vi "Setup SMU_PD and Measure Capacitance Only - Copy.vi"(0 "Semiconductor Module Context":T2, 1 "SMU_PD_Pin":string[](array[string])=["VDD"], 2 "Measurement Id":string="CMax", 3 "PD_v":dbl=41.0 format="%#_13g", 5 "error in (no error)":errorcluster, 6 "VNAs Measurement Parameters":T1) -> (14 "Semiconductor Module Context Out":T2, 19 "error out":errorcluster)   [LabVIEW 2013]
uses:
  <vilib>/NI_TestStand_SemiconductorModule/NI_TestStand_Semiconductor_Module.lvlibp/PinMap/General/SemiconductorModuleContext.ctl
  VNA/VNAs Measurement Parameters.ctl
  <vilib>/NI_TestStand_SemiconductorModule/NI_TestStand_Semiconductor_Module.lvlibp
panel:
  in  "SMU_PD_PU_v":dbl=1.8 caption="voltage level" format="%_6p"
  in  "SMU_PD_PU_Pin":string[](array[string])=["VDD"]
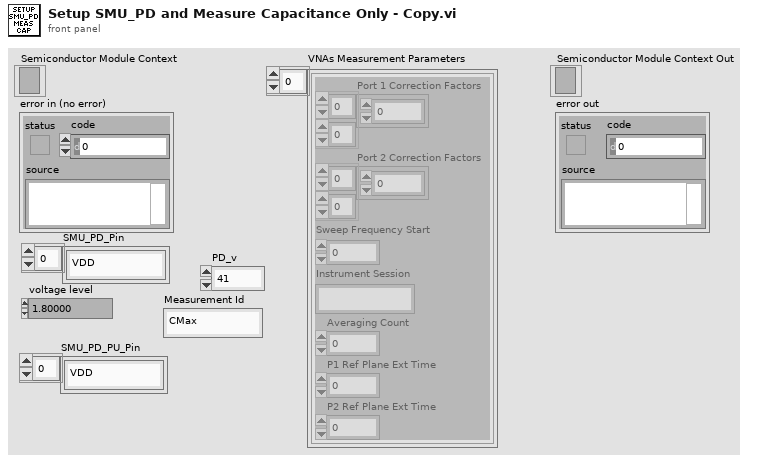
[diagram p1: front panel]
types:
  T1 = typedef "VNAs Measurement Parameters.ctl" = cluster{"Port 1 Correction Factors":cdb[][], "Port 2 Correction Factors":cdb[][], "Sweep Frequency Start":dbl, "Instrument Session":string, "Averaging Count":i32, "P1 Ref Plane Ext Time":dbl, "P2 Ref Plane Ext Time":dbl}[]
  T2 = typedef "NI_TestStand_Semiconductor_Module.lvlibp/SemiconductorModuleContext.ctl" = refnum<k7>
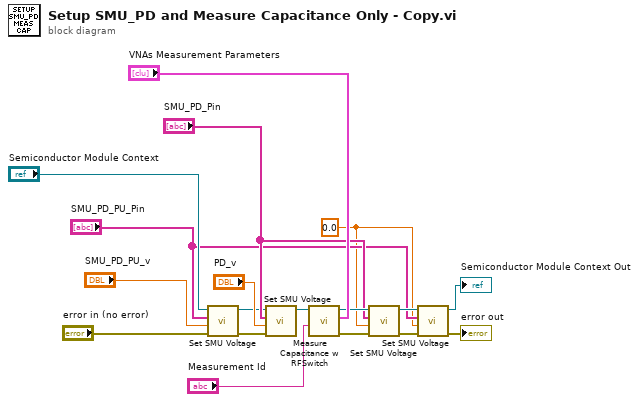
[diagram p0: block diagram]
diagram:
  w1 = 0.0 ("VDD voltage level")
  n1 = call "Set SMU Voltage.vi"("error in (no error)"="error in (no error)", "VDD voltage level"="SMU_PD_PU_v", "Pins"="SMU_PD_PU_Pin", "Semiconductor Module Context"="Semiconductor Module Context") -> ("error out"=w10:errorcluster, "Semiconductor Module Context Out"=w6:T2)  [unwired: 5 in, 1 out]
  n2 = call "Set SMU Voltage.vi"("error in (no error)"=w10, "VDD voltage level"="PD_v", "Pins"="SMU_PD_Pin", "Semiconductor Module Context"=w6) -> ("Semiconductor Module Context Out"=w12:T2)  [unwired: 5 in, 2 out]
  n3 = call "Measure Capacitance w RFSwitch.vi"("VNAs Measurement Parameters"="VNAs Measurement Parameters", "Measurement Id"="Measurement Id", "Semiconductor Module Context"=w12) -> ("error out"=w13:errorcluster, "Semiconductor Module Context Out"=w15:T2)  [unwired: 6 in, 1 out]
  n4 = call "Set SMU Voltage.vi"("error in (no error)"=w13, "VDD voltage level"=w1, "Pins"="SMU_PD_Pin", "Semiconductor Module Context"=w15) -> ("error out"=w9:errorcluster, "Semiconductor Module Context Out"=w5:T2)  [unwired: 5 in, 1 out]
  n5 = call "Set SMU Voltage.vi"("error in (no error)"=w9, "VDD voltage level"=w1, "Pins"="SMU_PD_PU_Pin", "Semiconductor Module Context"=w5) -> ("error out"=→"error out":errorcluster, "Semiconductor Module Context Out"=→"Semiconductor Module Context Out":T2)  [unwired: 5 in, 1 out]
